vi "Run Help Window.vi"(8 "error in (no error)":errorcluster) -> (0 "error out":errorcluster)   [LabVIEW 2017]
doc: "Starts <b>Help Window</b> asynchronous call (and forget)."
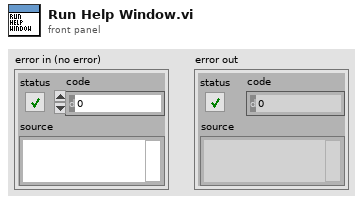
[diagram p1: front panel]
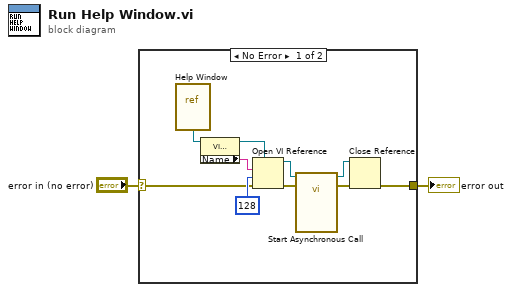
[diagram p0: block diagram]
diagram:
  n1 = case shown="No Error" "error in (no error)" {
    selector: "error in (no error)" -> [w3 w13]
    tunnel: [w4 w13] -> w2
    frame No Error {
      n2 = vi-ref "Help Window.vi"() -> (w8:refnum<vi>)
      n3 = property class="VI (strict)"(reference=w8) -> (reference out=w12:refnum<vi>, "Name"=w5:string)  [unwired: 1 in, 1 out]
      n4 = Open VI Reference(type specifier VI Refnum (for type only)=w12, vi path=w5, options=128, error in (no error)=w3) -> (vi reference=w7:refnum<vi>, error out=w9:errorcluster)  [unwired: 2 in]
      n5 = call-by-ref "Start Asynchronous Call"(reference=w7, error in=w9) -> (reference out=w11:refnum<vi>, error out=w10:errorcluster)  [unwired: 12 in]
      n6 = Close Reference(reference=w11, error in (no error)=w10) -> (error out=w4:errorcluster)
    }
    frame Error {
    }
  }
  "error out" <- w2
